vi "Helmholtz2D_Cal RHS_Apply BC.vi"(10 "Boundary Condition":cluster{"type":T1, "Value":dbl[]}[](array[cluster]) {"type" items=["Dirichlet", "Neumann"]}, 11 "RHS In":dbl[](array[numeric])) -> (3 "RHS Out":dbl[](array[numeric]))   [LabVIEW 2020, in "NI_PDE.lvlib"]
uses:
  <vilib>/gmath/NI_PDE.lvlib
  <vilib>/gmath/pde.llb/Common/PDE_BC Type.ctl
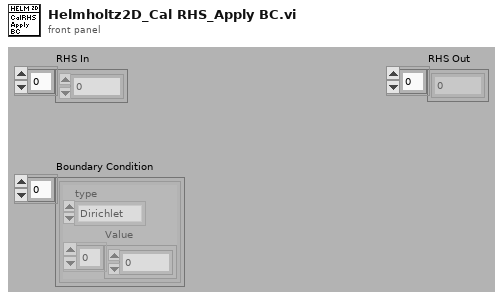
[diagram p1: front panel]
types:
  T1 = typedef "NI_PDE.lvlib/PDE_BC Type.ctl" = i32
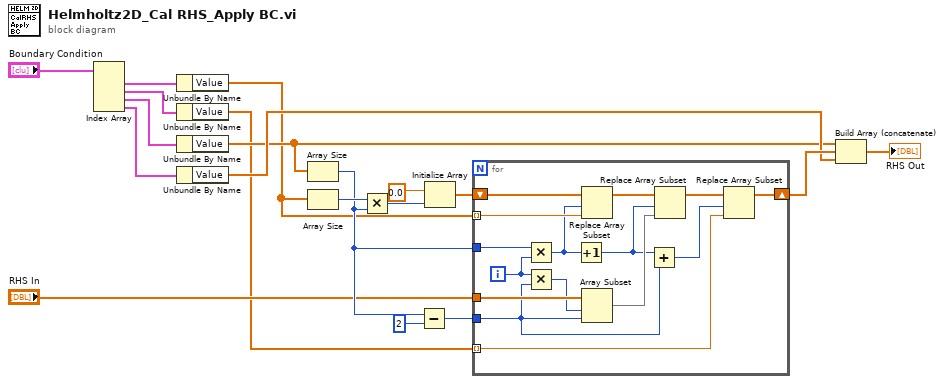
[diagram p0: block diagram]
diagram:
  n1 = Index Array(array="Boundary Condition") -> (element #1=w8:cluster{"type":T1, "Value":dbl[]}, element #2=w7:cluster{"type":T1, "Value":dbl[]}, element #3=w6:cluster{"type":T1, "Value":dbl[]}, element #4=w5:cluster{"type":T1, "Value":dbl[]})  [unwired: 4 in]
  n2 = Unbundle By Name(w8) -> ("Value"=w2:dbl[])
  n3 = Unbundle By Name(w7) -> ("Value"=w1:dbl[])
  n4 = Unbundle By Name(w6) -> ("Value"=w3:dbl[])
  n5 = Unbundle By Name(w5) -> ("Value"=w4:dbl[])
  n6 = Array Size(array=w3) -> (size(s)=w15:i32)
  n7 = Array Size(array=w2) -> (size(s)=w18:i32)
  n8 = Multiply(x=w18, y=w15) -> (x*y=w17:i32)
  n9 = Subtract(x=w15, y=2) -> (x-y=w13:i32)
  n10 = Initialize Array(0.0 ("element"), w17) -> (w16:dbl[])
  n11 = for {
    tunnel: w2 -> [w32] mode=indexing
    tunnel: w1 -> [w24] mode=indexing
    shift-right: [w21] -> w12
    shift-left: w16 -> [w34]
    tunnel: "RHS In" -> [w29]
    tunnel: w15 -> [w33]
    tunnel: w13 -> [w20]
    i -> [w27]
    n12 = Multiply(x=w33, y=w27) -> (x*y=w30:i32)
    n13 = Multiply(x=w27, y=w20) -> (x*y=w26:i32)
    n14 = Increment(x=w30) -> (x+1=w23:i32)
    n15 = Replace Array Subset(array=w34, new element=w32, index=w30) -> (w31:dbl[])
    n16 = Array Subset(array=w29, index=w26, length=w20) -> (w28:dbl[])
    n17 = Add(x=w23, y=w20) -> (x+y=w22:i32)
    n18 = Replace Array Subset(array=w31, new element=w28, index=w23) -> (w25:dbl[])
    n19 = Replace Array Subset(array=w25, new element=w24, index=w22) -> (w21:dbl[])
  }
  n20 = Build Array (concatenate)(w3, w12, w4) -> (→"RHS Out":dbl[])
